vi "write out sonde data.vi"(5 "data column offset":i32, 6 "Sonde Data Cluster":T1 caption="Cluster" {"Salinity" format="%_3g"; "Temp deg C" format="%_2g"; "ORP" format="%_4g"; "pH" format="%_4g"; "Dissolved\nOxygen mg/L" format="%_4g"; "Specific\nCond (mS)" format="%_4g"; "Cumulative\nVolume (ml)" format="%#_4g"}, 7 "start of last occupied row":cluster{"row":i32, "column":i32}, 8 "error in (no error)":errorcluster, 9 "Row Offset":i32, 10 "Header data columns":i32[](array[numeric]), 11 "NI_report in":refnum<class "NI_report.lvclass">) -> (0 "error out":errorcluster, 3 "NI_report out":refnum<class "NI_report.lvclass">)   [LabVIEW 2016]
uses:
  <vilib>/Utility/NIReport.llb/NI_report.lvclass
  sonde cluster.ctl
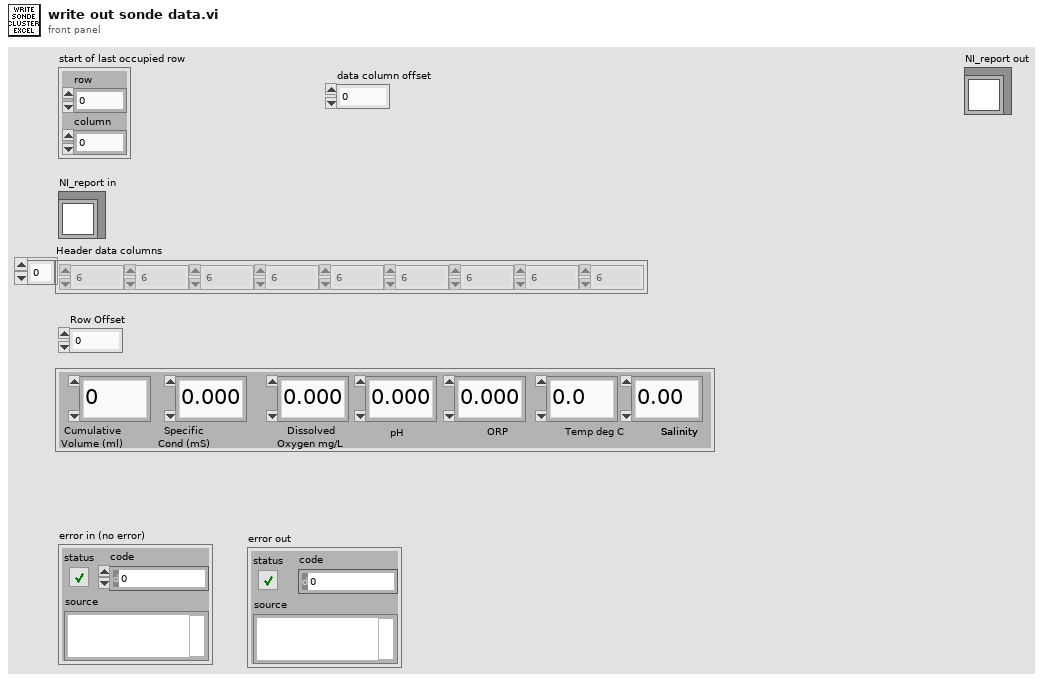
[diagram p1: front panel]
types:
  T1 = typedef "sonde cluster.ctl" = cluster{"Cumulative\nVolume (ml)":dbl, "Specific\nCond (mS)":dbl, "Dissolved\nOxygen mg/L":dbl, "pH":dbl, "ORP":dbl, "Temp deg C":dbl, "Salinity":dbl}
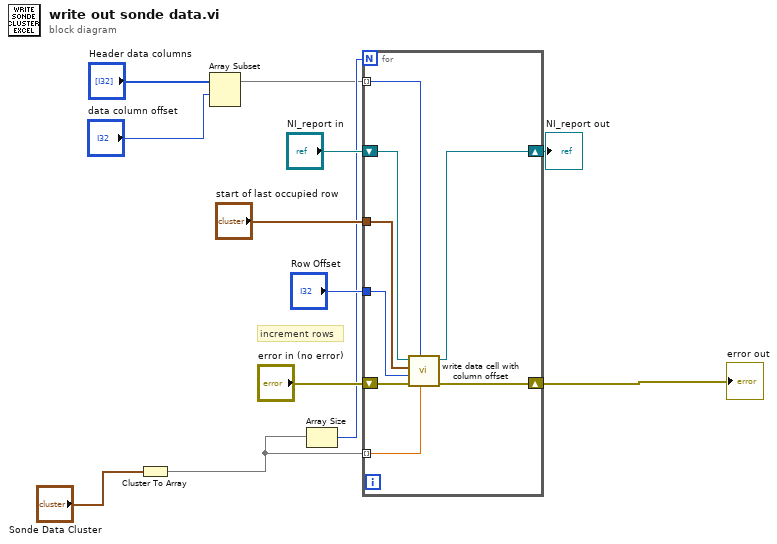
[diagram p0: block diagram]
diagram:
  # "increment rows"
  n1 = Cluster To Array(cluster="Sonde Data Cluster") -> (array=w1:dbl[])
  n2 = Array Subset(array="Header data columns", index="data column offset") -> (w3:i32[])  [unwired: 1 in]
  n3 = Array Size(array=w1) -> (size(s)=w6:i32)
  n4 = for {
    N: w6 -> [_]
    tunnel: "start of last occupied row" -> [w18]
    tunnel: "Row Offset" -> [w17]
    tunnel: w3 -> [w13] mode=indexing
    shift-right: [w16] -> w11
    shift-left: "error in (no error)" -> [w20]
    shift-right: [w15] -> w12
    shift-left: "NI_report in" -> [w19]
    tunnel: w1 -> [w14] mode=indexing
    n5 = call "write data cell with column offset.vi"("Data Input"=w14, "data column"=w13, "error in (no error)"=w20, "row offset"=w17, "start of last occupied row"=w18, "NI_report in"=w19) -> ("error out"=w16:errorcluster, "NI_report out"=w15:refnum<class "NI_report.lvclass">)  [unwired: 4 in]
  }
  "NI_report out" <- w12
  "error out" <- w11
